vi "Polar Plots.vi"() -> ()   [LabVIEW 2011]
uses:
  <vilib>/Heliosphere Research LLC/Advanced Plotting Toolkit/Advanced Plotting Toolkit.lvlib
  <vilib>/Heliosphere Research LLC/Advanced Plotting Toolkit/api_annotations/LegendPositions.ctl
  <vilib>/Heliosphere Research LLC/Advanced Plotting Toolkit/api_core/NewPlotType.ctl
panel:
  in  "Plot Type":T1=enum."Polar Axes"
  out "Polar Plot":picture
  # "Polar Plots"
  # "There is no special \"Polar API\" for making polar plots with the\nToolkit.  Instead, we specify polar axes when creating the plot,\nand then use the normal 1D plotting VIs like Line.vi, Scatter.vi\nor Bar.vi.\n\nThis example shows a two datasets (line and scatter) along with\na legend, displayed on polar axes.  All you have to do to\nswitch back and forth between polar and rectangular axes is\nchange the \"Plot Type\" input to New.vi.  The Toolkit figures\neverything else out.\n\nTry changing the Plot Type below to Rectangular.\n\nNote that for polar plots, you specify the X (theta) positions in\nradians rather than degrees."
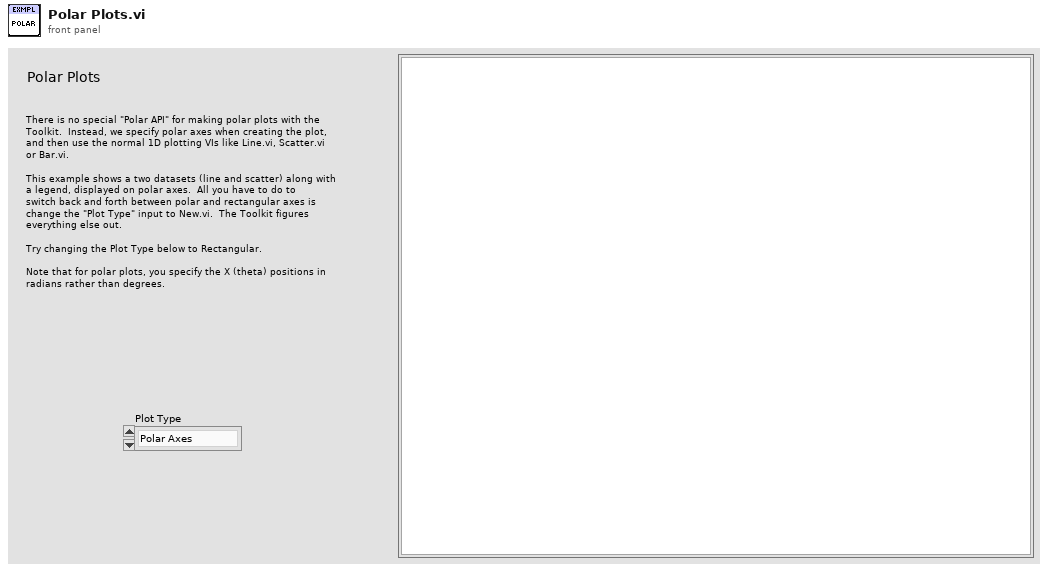
[diagram p1: front panel]
types:
  T1 = typedef "Advanced Plotting Toolkit.lvlib/NewPlotType.ctl" = enum16{"Rectangular Axes", "Polar Axes"}
  T2 = typedef "Advanced Plotting Toolkit.lvlib/LegendPositions.ctl" = enum16{"Default", "Top Right", "Top", "Top Left", "Left", "Bottom Left", "Bottom", "Bottom Right", "Right", "Center"}
  T3 = typedef "Advanced Plotting Toolkit.lvlib/PlotID.ctl" = i32
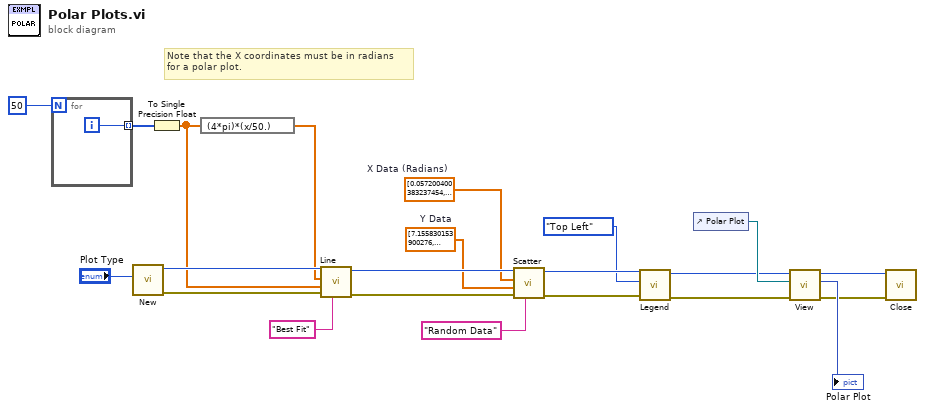
[diagram p0: block diagram]
diagram:
  w2 = dbl[] [7.155830153900276, 9.542188876131137, 12.964694396849413, 9.608341141823788, 6.1353360563741886, 6.30777678828452, 3.492719738169233, 10.475116986030116, 11.73663627292205, 9.491795162093482, 7.728614897569347, 7.364294454741597, 8.119284592814168, 15.797279906006743, 17.877027122762485, 9.872453803456173, 11.92676816224991, 11.544417787449923, 13.355029071220148, 11.004738904107189, 18.9948333312404, 10.21061640353804, 17.296824052448397, 18.638122987745824, 10.709910178352452, 19.10439454078672, 19.787382610027898, 11.327541441866765, 14.241158033621998, 22.07915169723564, 17.76078678939979, 15.762869387274339, 15.57550201850206, 21.792615537623313, 19.784850956025274, 17.130940096933983, 18.3794433426299, 21.311416124980916, 21.059843733367853, 21.95540285013855, 20.301233212792503, 24.7544069142969, 18.007661210833255, 22.570156237910933, 22.09117440707828, 25.097583520899626, 20.564812672267127, 23.0196482170539, 21.200137713273307, 22.4535930398079, 27.793943822024197, 32.78641772203316, 23.74509687361215, 28.577157826330463, 26.6708925326644, 26.1109635866, 26.617534907693774, 34.15668722579318, 25.46491758886637, 35.235767241238314, 29.554319135183146, 24.942815835796036, 35.62822844966281, 31.049128110077945, 25.548272771674718, 26.235311637411193, 34.15630727207706, 35.77745806166092, 38.95898597399431, 32.806395796984454, 37.63006019937063, 31.808189701468205, 35.01126180391481, 34.56957433052476, 34.028597640107684, 32.151213309973805, 35.87583950029433, 32.72613016447266, 31.82053098004376, 33.28715657829349, 39.27026312080221, 32.427077901713645, 35.75721114771309, 42.34616052367428, 36.00573325275944, 41.28471226095021, 44.09978366560297, 44.96319270520742, 35.69838521869672, 45.81049241320639, 41.798198783692456, 39.49939714307897, 37.39275979621768, 46.82600394250823, 47.66645927999525, 42.07724620361945, 43.749041566804166, 41.935197302594325, 41.54983842391538, 38.895016801326435]  # Y Data
  w10 = dbl[] [0.057200400383237454, 1.932873052543739, 0.28768326582210346, 1.8073323231744194, 0.9674781382959977, 2.92047258964459, 2.3821559070735905, 3.4218770450040847, 1.9853703106669958, 1.2082317552286732, 4.012400323953288, 3.08128142045082, 1.2133644338050165, 3.848769147310155, 1.5770212460583501, 4.402161319157912, 2.0261266598920855, 2.7606789492136445, 2.543484217647808, 4.1829475547827375, 2.026581294288934, 5.03621106420812, 3.0755942019939178, 3.7733475997545467, 4.302014531833393, 4.382846829969237, 4.842139009809148, 4.8092417099587115, 2.882298114601737, 3.382057920523399, 3.4037660911028857, 5.96983385273861, 3.1724565362676325, 4.476931239041165, 5.230298315752474, 5.334284423363629, 5.179310131551981, 6.520406177910641, 6.549004340792519, 4.4284533130862265, 4.587366936496216, 6.519644096566266, 5.270381871159589, 6.149419457696073, 7.2620751237705035, 5.015743270395747, 6.535348985444991, 6.146521344793193, 6.999258223047373, 6.225044848836166, 7.806785048539754, 7.199866081374925, 7.991046522721868, 6.594376498090614, 5.173395189752654, 5.745837084867013, 8.414902042703526, 7.45036006053253, 7.37133947514793, 7.3113200500656745, 6.446611825051214, 8.401553037813557, 7.4491216348152305, 8.93934465646939, 6.446748806480898, 6.2829244674494475, 7.605382888090498, 9.125444742161445, 9.525469587110084, 9.30779431268778, 9.587758842371551, 7.559722445012978, 7.443455178581228, 8.068196636219014, 8.583461569692245, 10.075376121860147, 7.28889449264635, 8.707436925809859, 7.932604623578424, 9.872977465196067, 10.36497642235918, 10.763579800206603, 9.711594253402556, 8.357271059141208, 8.13298138602365, 9.652183955447803, 10.971572785040824, 10.227072621262732, 8.660802585197759, 10.865159311316196, 10.035366497845722, 10.113798324466146, 10.253369857397061, 10.411806552725121, 11.120194666107965, 11.24102515549767, 9.333092160376292, 10.367714176179915, 9.501174420441641, 10.074882713265858]  # X Data (Radians)
  # "Note that the X coordinates must be in radians\nfor a polar plot."
  n1 = for {
    N: 50 -> [_]
    tunnel: [w23] -> w18 mode=indexing
    i -> [w23]
  }
  n2 = call <vilib>:"New.vi"("Plot Type"="Plot Type") -> ("error out"=w14:errorcluster, "Plot ID"=w17:T3)  [unwired: 9 in]
  n3 = To Single Precision Float(number=w18) -> (single precision float=w15:sgl[])
  n4 = expression code="(4*pi)*(x/50.)"(w15) -> (w16:sgl[])
  n5 = call <vilib>:"Line.vi"("Legend Title"="Best Fit", "error in (no error)"=w14, "Y Data"=w15, "X Data"=w16, "Plot ID"=w17) -> ("error out"=w11:errorcluster, "Plot ID out"=w12:T3)  [unwired: 5 in]
  n6 = call <vilib>:"Scatter.vi"("Legend Title"="Random Data", "error in (no error)"=w11, "Y Data"=w2, "X Data"=w10, "Plot ID"=w12) -> ("error out"=w5:errorcluster, "Plot ID Out"=w7:T3)  [unwired: 5 in]
  n7 = call <vilib>:"Legend.vi"("error in (no error)"=w5, "Position"=LegendPositions."Top Left", "Plot ID"=w7) -> ("error out"=w4:errorcluster, "Plot ID Out"=w6:T3)  [unwired: 7 in]
  n8 = control-ref of="Polar Plot"() -> (w22:refnum<vi>)
  n9 = call <vilib>:"View.vi"("error in (no error)"=w4, "Ref for Sizing"=w22, "Plot ID"=w6) -> ("error out"=w1:errorcluster, "Picture"=→"Polar Plot":picture, "Plot ID Out"=w20:T3)  [unwired: 6 in]
  n10 = call <vilib>:"Close.vi"("error in (no error)"=w1, "Plot ID"=w20) -> ()  [unwired: 9 in, 1 out]
